vi "Thin Etalon Linewidth Sweep 2.0.vi"(8 "Error In":errorcluster) -> (0 "Error Out":errorcluster, 1 "Done":bool, 2 "Time Elapsed":dbl, 3 "Center Position":i32, 4 "Lower Limit":i32, 5 "Upper Limit":i32)   [LabVIEW 2013]
panel:
  in  "Mode Jump Threshold":dbl=0.1
  in  "Sweep Step Speed (ms)":u32=10
  in  "Linewidth Threshold":dbl=1.1
  in  "Sweep Step Size":i32=2
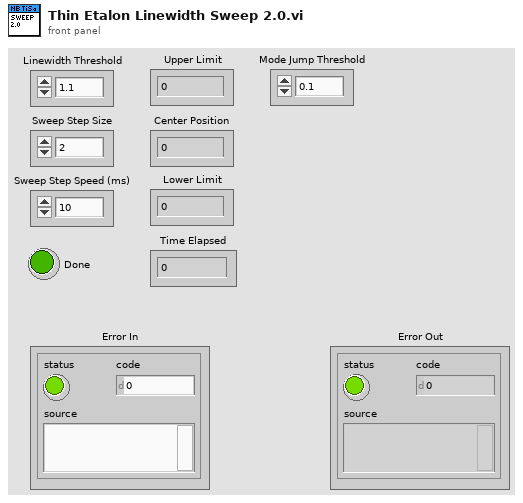
[diagram p1: front panel]
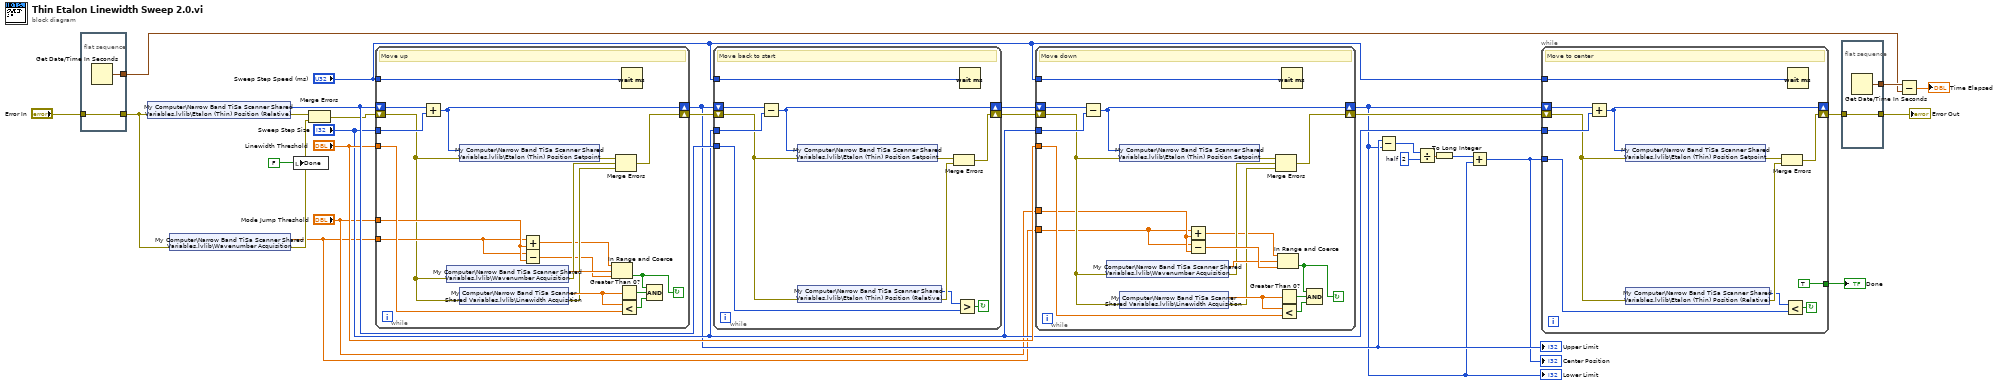
[diagram p0: block diagram]
diagram:
  w19 = 2  # half
  n1 = flat-sequence {
    tunnel: "Error In" -> [w31]
    tunnel: [w31] -> w3
    tunnel: [w30] -> w10
    frame #0 {
      n2 = Get Date/Time In Seconds() -> (seconds since 1Jan1904=w30:timestamp)
    }
  }
  n3 = shared-variable "My Computer\\Narrow Band TiSa Scanner Shared Variables.lvlib\\Etalon (Thin) Position (Relative)"(error in=w3) -> (w28:i32, error out=w4:errorcluster)
  n4 = shared-variable "My Computer\\Narrow Band TiSa Scanner Shared Variables.lvlib\\Wavenumber Acquisition"(error in=w3) -> (w1:dbl, error out=w6:errorcluster)
  n5 = local write "Done"(FALSE) -> ()
  n6 = Merge Errors(w4, w6) -> (w5:errorcluster)
  n7 = while {
    tunnel: "Sweep Step Size" -> [w49]
    shift-right: [w48] -> w20
    shift-left: w28 -> [w50]
    tunnel: "Linewidth Threshold" -> [w46]
    tunnel: "Sweep Step Speed (ms)" -> [w45]
    shift-right: [w44] -> w29
    shift-left: w5 -> [w33]
    tunnel: "Mode Jump Threshold" -> [w37]
    tunnel: w1 -> [w36]
    stop <- w32 continue-if-true
    # "Move up"
    n8 = Add(x=w50, y=w49) -> (x+y=w48:i32)
    n9 = shared-variable "My Computer\\Narrow Band TiSa Scanner Shared Variables.lvlib\\Wavenumber Acquisition"(error in=w33) -> (w42:dbl, error out=w41:errorcluster)
    n10 = shared-variable "My Computer\\Narrow Band TiSa Scanner Shared Variables.lvlib\\Etalon (Thin) Position Setpoint"(w48, error in=w33) -> (error out=w47:errorcluster)
    n11 = shared-variable "My Computer\\Narrow Band TiSa Scanner Shared Variables.lvlib\\Linewidth Acquisition"(error in=w33) -> (w43:dbl, error out=w40:errorcluster)
    n12 = Add(x=w36, y=w37) -> (x+y=w35:dbl)
    n13 = Subtract(x=w36, y=w37) -> (x-y=w34:dbl)
    n14 = In Range and Coerce(upper limit=w35, x=w42, lower limit=w34) -> (In Range?=w32:bool)  [unwired: 1 out]
    n15 = Merge Errors(w47, w41, w40) -> (w44:errorcluster)
    n16 = Greater Than 0?(x=w43) -> (x > 0?=w39:bool)
    n17 = Less?(x=w43, y=w46) -> (x < y?=w38:bool)
    n18 = Wait (ms)(milliseconds to wait=w45) -> ()  [unwired: 1 out]
    n19 = Compound Arithmetic op=AND(w32, w39, w38) -> ()  [unwired: 1 out]
  }
  "Upper Limit" <- w20
  n20 = while {
    tunnel: "Sweep Step Size" -> [w60]
    shift-right: [w59] -> w27
    shift-left: w20 -> [w61]
    tunnel: w28 -> [w54]
    tunnel: "Sweep Step Speed (ms)" -> [w53]
    shift-right: [w51] -> w26
    shift-left: w29 -> [w52]
    stop <- w55 continue-if-true
    # "Move back to start"
    n21 = Subtract(x=w61, y=w60) -> (x-y=w59:i32)
    n22 = shared-variable "My Computer\\Narrow Band TiSa Scanner Shared Variables.lvlib\\Etalon (Thin) Position Setpoint"(w59, error in=w52) -> (error out=w58:errorcluster)
    n23 = shared-variable "My Computer\\Narrow Band TiSa Scanner Shared Variables.lvlib\\Etalon (Thin) Position (Relative)"(error in=w52) -> (w56:i32, error out=w57:errorcluster)
    n24 = Merge Errors(w58, w57) -> (w51:errorcluster)
    n25 = Greater?(x=w56, y=w54) -> (0:w55:bool)
    n26 = Wait (ms)(milliseconds to wait=w53) -> ()  [unwired: 1 out]
  }
  n27 = while {
    tunnel: "Sweep Step Size" -> [w79]
    shift-right: [w78] -> w15
    shift-left: w27 -> [w80]
    tunnel: "Linewidth Threshold" -> [w76]
    tunnel: "Sweep Step Speed (ms)" -> [w75]
    shift-right: [w74] -> w24
    shift-left: w26 -> [w72]
    tunnel: "Mode Jump Threshold" -> [w64]
    tunnel: w1 -> [w63]
    stop <- w62 continue-if-true
    # "Move down"
    n28 = Subtract(x=w80, y=w79) -> (x-y=w78:i32)
    n29 = shared-variable "My Computer\\Narrow Band TiSa Scanner Shared Variables.lvlib\\Wavenumber Acquisition"(error in=w72) -> (w70:dbl, error out=w69:errorcluster)
    n30 = shared-variable "My Computer\\Narrow Band TiSa Scanner Shared Variables.lvlib\\Etalon (Thin) Position Setpoint"(w78, error in=w72) -> (error out=w77:errorcluster)
    n31 = shared-variable "My Computer\\Narrow Band TiSa Scanner Shared Variables.lvlib\\Linewidth Acquisition"(error in=w72) -> (w73:dbl, error out=w68:errorcluster)
    n32 = Add(x=w63, y=w64) -> (x+y=w67:dbl)
    n33 = Subtract(x=w63, y=w64) -> (x-y=w71:dbl)
    n34 = Merge Errors(w77, w69, w68) -> (w74:errorcluster)
    n35 = In Range and Coerce(upper limit=w67, x=w70, lower limit=w71) -> (In Range?=w62:bool)  [unwired: 1 out]
    n36 = Greater Than 0?(x=w73) -> (x > 0?=w66:bool)
    n37 = Less?(x=w73, y=w76) -> (x < y?=w65:bool)
    n38 = Wait (ms)(milliseconds to wait=w75) -> ()  [unwired: 1 out]
    n39 = Compound Arithmetic op=AND(w62, w66, w65) -> ()  [unwired: 1 out]
  }
  "Lower Limit" <- w15
  n40 = Subtract(x=w20, y=w15) -> (x-y=w21:i32)
  n41 = Divide(x=w21, y=w19) -> (x/y=w18:dbl)
  n42 = To Long Integer(number=w18) -> (32bit integer=w14:i32)
  n43 = Add(x=w14, y=w15) -> (x+y=w13:i32)
  "Center Position" <- w13
  n44 = while {
    tunnel: "Sweep Step Size" -> [w91]
    shift-right: [w90] -> _
    shift-left: w15 -> [w92]
    tunnel: w13 -> [w85]
    tunnel: "Sweep Step Speed (ms)" -> [w84]
    shift-right: [w82] -> w12
    shift-left: w24 -> [w83]
    tunnel: [TRUE] -> w17
    stop <- w86 continue-if-true
    # "Move to center"
    n45 = Add(x=w92, y=w91) -> (x+y=w90:i32)
    n46 = shared-variable "My Computer\\Narrow Band TiSa Scanner Shared Variables.lvlib\\Etalon (Thin) Position Setpoint"(w90, error in=w83) -> (error out=w89:errorcluster)
    n47 = shared-variable "My Computer\\Narrow Band TiSa Scanner Shared Variables.lvlib\\Etalon (Thin) Position (Relative)"(error in=w83) -> (w87:i32, error out=w88:errorcluster)
    n48 = Merge Errors(w89, w88) -> (w82:errorcluster)
    n49 = Less?(x=w87, y=w85) -> (x < y?=w86:bool)
    n50 = Wait (ms)(milliseconds to wait=w84) -> ()  [unwired: 1 out]
  }
  "Done" <- w17
  n51 = flat-sequence {
    tunnel: w12 -> [w93]
    tunnel: [w94] -> w11
    tunnel: [w93] -> w7
    frame #0 {
      n52 = Get Date/Time In Seconds() -> (seconds since 1Jan1904=w94:timestamp)
    }
  }
  n53 = Subtract(x=w11, y=w10) -> (x-y=→"Time Elapsed":dbl)
  "Error Out" <- w7
